vi "delayTransmax.vi"(8 "error in (no error)":errorcluster, 9 "Toffset":dbl=1.5 format="%#_13g", 10 "Tmax":dbl, 11 "Bcount":i32) -> (0 "error out":errorcluster, 3 "Tdelay":dbl)   [LabVIEW 2018]
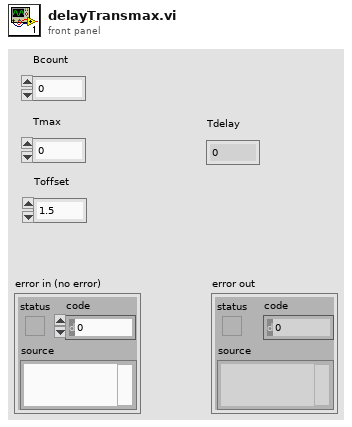
[diagram p1: front panel]
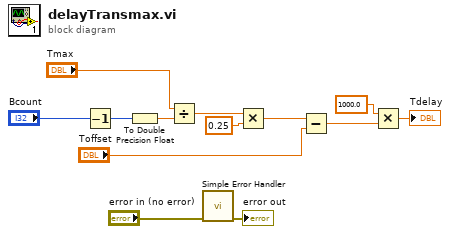
[diagram p0: block diagram]
diagram:
  n1 = Decrement(x="Bcount") -> (x-1=w5:i32)
  n2 = To Double Precision Float(number=w5) -> (double precision float=w6:dbl)
  n3 = Divide(x="Tmax", y=w6) -> (x/y=w7:dbl)
  n4 = call <vilib>:"Simple Error Handler.vi"("error in (no error)"="error in (no error)") -> ("error out"=→"error out":errorcluster)  [unwired: 4 in, 4 out]
  n5 = Multiply(x=w7, y=0.25) -> (x*y=w4:dbl)
  n6 = Subtract(x=w4, y="Toffset") -> (x-y=w3:dbl)
  n7 = Multiply(x=1000.0, y=w3) -> (x*y=→"Tdelay":dbl)
